vi "DaysInMonthSubVI.vi"(1 "Year":i16 min=0 step=1, 2 "Month":i8=1 min=1 max=12 step=1) -> (0 "Max Days in Month":dbl)   [LabVIEW 2020]
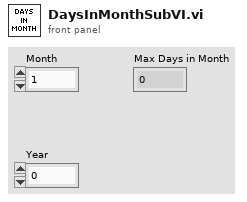
[diagram p1: front panel]
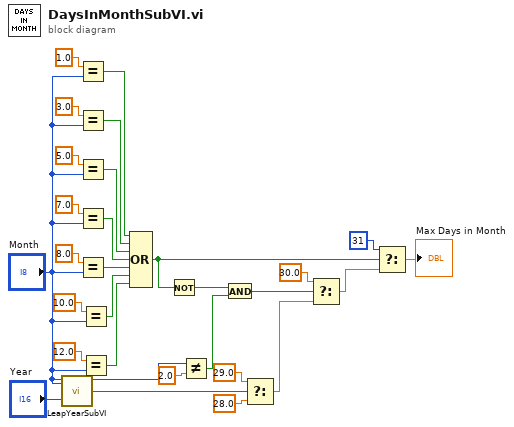
[diagram p0: block diagram]
diagram:
  n1 = call "LeapYearSubVI.vi"("Year"="Year", "Month"="Month") -> ("Leap Year?"=w11:bool)
  n2 = Equal?(x=1.0, y="Month") -> (x = y?=w8:bool)
  n3 = Equal?(x=3.0, y="Month") -> (x = y?=w7:bool)
  n4 = Equal?(x=5.0, y="Month") -> (x = y?=w6:bool)
  n5 = Equal?(x=7.0, y="Month") -> (x = y?=w5:bool)
  n6 = Equal?(x=8.0, y="Month") -> (x = y?=w4:bool)
  n7 = Equal?(x=10.0, y="Month") -> (x = y?=w3:bool)
  n8 = Equal?(x=12.0, y="Month") -> (x = y?=w2:bool)
  n9 = Compound Arithmetic op=OR(w8, w7, w6, w5, w4, w3, w2) -> (w1:bool)
  n10 = Not(x=w1) -> (.not. x?=w24:bool)
  n11 = Not Equal?(x="Month", y=2.0) -> (x != y?=w26:bool)
  n12 = And(x=w24, y=w26) -> (x .and. y?=w28:bool)
  n13 = Select(t=29.0, s=w11, f=28.0) -> (s? t:f=w27:dbl)
  n14 = Select(t=30.0, s=w28, f=w27) -> (s? t:f=w22:dbl)
  n15 = Select(t=31, s=w1, f=w22) -> (s? t:f=→"Max Days in Month":dbl)
